vi "Disconnect Channels.vi"(8 "error in (no error)":errorcluster, 9 "Deleted Channels":refnum<class "TBM channel.lvclass">[](array[class]), 10 "instance id":string, 11 "Engine Configuration in":refnum<class "engine configuration.lvclass">) -> (0 "error out":errorcluster, 3 "Engine Configuration out":refnum<class "engine configuration.lvclass">)   [LabVIEW 2013, in "tag bus configurable plugin editor node.lvclass"]
uses:
  tag bus configurable plugin editor node.lvclass
  <vilib>/NI/Tag Bus Module Framework/channel/TBM channel.lvclass
  <vilib>/NI/Module Execution Interface/Engine Configuration/engine configuration.lvclass
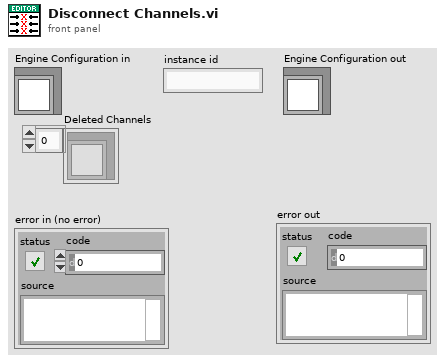
[diagram p1: front panel]
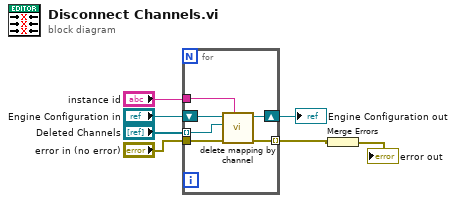
[diagram p0: block diagram]
diagram:
  n1 = for {
    tunnel: "Deleted Channels" -> [w13] mode=indexing
    tunnel: "error in (no error)" -> [w12]
    tunnel: [w9] -> w2 mode=indexing
    tunnel: "instance id" -> [w8]
    shift-right: [w10] -> w4
    shift-left: "Engine Configuration in" -> [w11]
    n2 = call <vilib>:"delete mapping by channel.vi"("owner ID"=w8, "error in"=w12, "channel"=w13, "engine configuration in"=w11) -> ("error out"=w9:errorcluster, "engine configuration out"=w10:refnum<class "engine configuration.lvclass">)  [unwired: 6 in]
  }
  "Engine Configuration out" <- w4
  n3 = Merge Errors(w2) -> (→"error out":errorcluster)
